vi "Enable Termnal Icon View(冲突时的文件备份2013-05-03 09-42-16).vi"   [LabVIEW 2012]
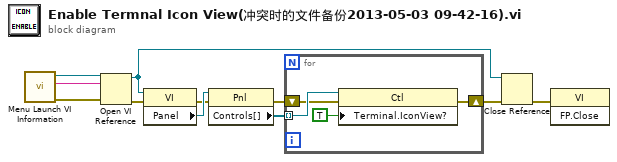
[diagram p0: block diagram]
diagram:
  n1 = call <vilib>:"Menu Launch VI Information.vi"() -> ("error out"=w3:errorcluster, "Menu Launch:VI"=w1:string, "Menu Launch:App"=w2:refnum<vi>)  [unwired: 9 in]
  n2 = Open VI Reference(application reference (local)=w2, vi path=w1, error in (no error)=w3) -> (vi reference=w5:refnum<vi>, error out=w9:errorcluster)  [unwired: 3 in]
  n3 = property class="VI"(reference=w5, error in=w9) -> (error out=w8:errorcluster, "Panel"=w11:refnum<vi>)  [unwired: 1 out]
  n4 = property class="Pnl"(reference=w11, error in=w8) -> (error out=w7:errorcluster, "Controls[]"=w10:refnum<vi>[])  [unwired: 1 out]
  n5 = for {
    tunnel: w10 -> [w15] mode=indexing
    shift-right: [w12] -> w6
    shift-left: w7 -> [w13]
    n6 = property class="Ctl"(reference=w15, error in=w13, "Terminal.IconView?"=TRUE ("接线端.图标视图？")) -> (error out=w12:errorcluster)  [unwired: 1 out]
  }
  n7 = Close Reference(reference=w5, error in (no error)=w6) -> (error out=w4:errorcluster)
  n8 = invoke class="VI" method="FP.Close"(error in=w4) -> ()  [unwired: 2 in, 3 out]
